vi "ASI_serialMove setpoint.vi"(0 "Axis":string, 1 "setpoint":i32, 2 "error in (no error)":errorcluster, 3 "VISA resource name":refnum<visa-resource-name>="COM7") -> (7 "error out":errorcluster)   [LabVIEW 2015]
doc: "Establishes connection with configured port (default = COM1).\nSends command MOVE X=x Y=y where x and y are integers denoting 10ths of a micron.\nSub-VI SerialWaitForStatusN.vi polls controller with STATUS command until 'N' (not busy) status is returned, or until a configured maximum number of unsuccessful tries (default = 400).\nDisconnects from configured port."
uses:
  <vilib>/Instr/_visa.llb/VISA Flush IO Buffer Mask.ctl
  Instance           1 20Saved   SerialMoveXY .vi
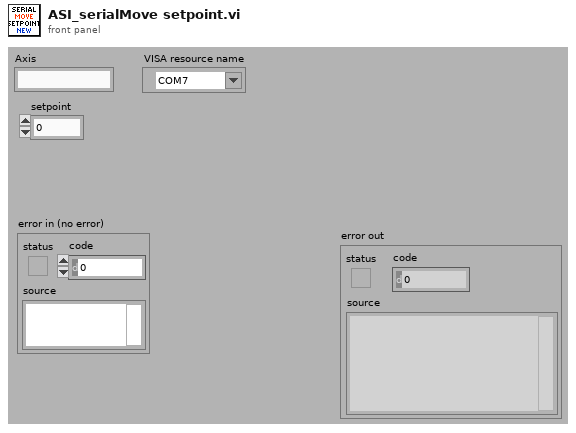
[diagram p1: front panel]
types:
  T1 = typedef "VISA Flush IO Buffer Mask.ctl" = u16
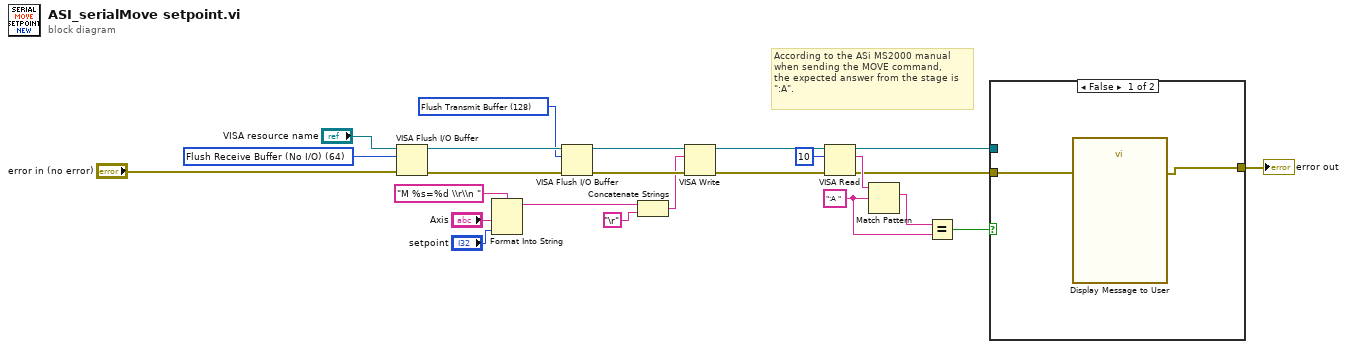
[diagram p0: block diagram]
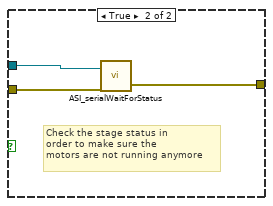
[diagram p2: hidden frame]
diagram:
  w13 = T1 128 items=["Flush Receive Buffer"=16, "Write Transmit Buffer to Device"=32, "Flush Receive Buffer (No I/O)"=64, "Flush Transmit Buffer"=128] ("Mask")
  w16 = T1 64 items=["Flush Receive Buffer"=16, "Write Transmit Buffer to Device"=32, "Flush Receive Buffer (No I/O)"=64, "Flush Transmit Buffer"=128] ("Mask")
  w4 = ":A " ("y")
  # "According to the ASi MS2000 manual\nwhen sending the MOVE command, \nthe expected answer from the stage is\n\":A\"."
  n1 = VISA Flush I/O Buffer(VISA resource name="VISA resource name", mask (16)=w16, error in (no error)="error in (no error)") -> (VISA resource name out=w14:refnum<visa-resource-name>, error out=w15:errorcluster)
  n2 = Format Into String "Format Into String"(format string="M %s=%d \\r\\n ", "Axis", "setpoint") -> (resulting string=w9:string)  [unwired: 2 in, 1 out]
  n3 = VISA Flush I/O Buffer(VISA resource name=w14, mask (16)=w13, error in (no error)=w15) -> (VISA resource name out=w11:refnum<visa-resource-name>, error out=w12:errorcluster)
  n4 = Concatenate Strings(w9, "\r") -> (w7:string)
  n5 = VISA Write(VISA resource name=w11, write buffer=w7, error in (no error)=w12) -> (VISA resource name out=w22:refnum<visa-resource-name>, error out=w10:errorcluster)  [unwired: 1 out]
  n6 = VISA Read(VISA resource name=w22, byte count=u32 10, error in (no error)=w10) -> (VISA resource name out=w19:refnum<visa-resource-name>, read buffer=w6:string, error out=w2:errorcluster)  [unwired: 1 out]
  n7 = Match Pattern(string=w6, regular expression=w4) -> (match substring=w5:string)  [unwired: 1 in, 3 out]
  n8 = Equal?(x=w5, y=w4) -> (x = y?=w20:bool)
  n9 = case shown="False" w20 {
    tunnel: w19 -> [_ w28]
    tunnel: [w25 w29] -> w1
    tunnel: w2 -> [w26 w27]
    frame False {
      n10 = call "Display Message to User"("error in (no error)"=w26) -> ("error out"=w25:errorcluster)  [unwired: 9 in, 1 out]
    }
    frame True {
      # "Check the stage status in\norder to make sure the \nmotors are not running anymore"
      n11 = call "ASI_serialWaitForStatus.vi"("error in"=w27, "VISA resource name"=w28) -> ("error out"=w29:errorcluster)  [unwired: 1 in]
    }
  }
  "error out" <- w1
